vi "Update Properties in SysDef.vi"(8 "error in (no error)":errorcluster, 10 "Changed Properties":T1[](array[typedef]), 11 "Node Ptr":T2 format="%.0x") -> (0 "error out":errorcluster, 3 "Item Ref out":T2 format="%.0x")   [LabVIEW 2017]
doc: "Check which property value was changed and update that."
uses:
  SLSC EDS API/JSON parsing/property.ctl
  <vilib>/NI Veristand/Custom Device API/Custom Device API.lvlib
  Shared/Constants.vi
  Shared/SLSC EDS Shared.lvlib
  <vilib>/NI Veristand/Custom Device API/Set Item Property (Variant).vi
  <vilib>/NI Veristand/Custom Device API/Get Item Property (Variant).vi
  SLSC EDS API/JSON parsing/propertySysDefPage.ctl
  <vilib>/NI Veristand/Custom Device API/Custom Device Item Ref.ctl
panel:
  out "Properties":T1[](array[typedef])
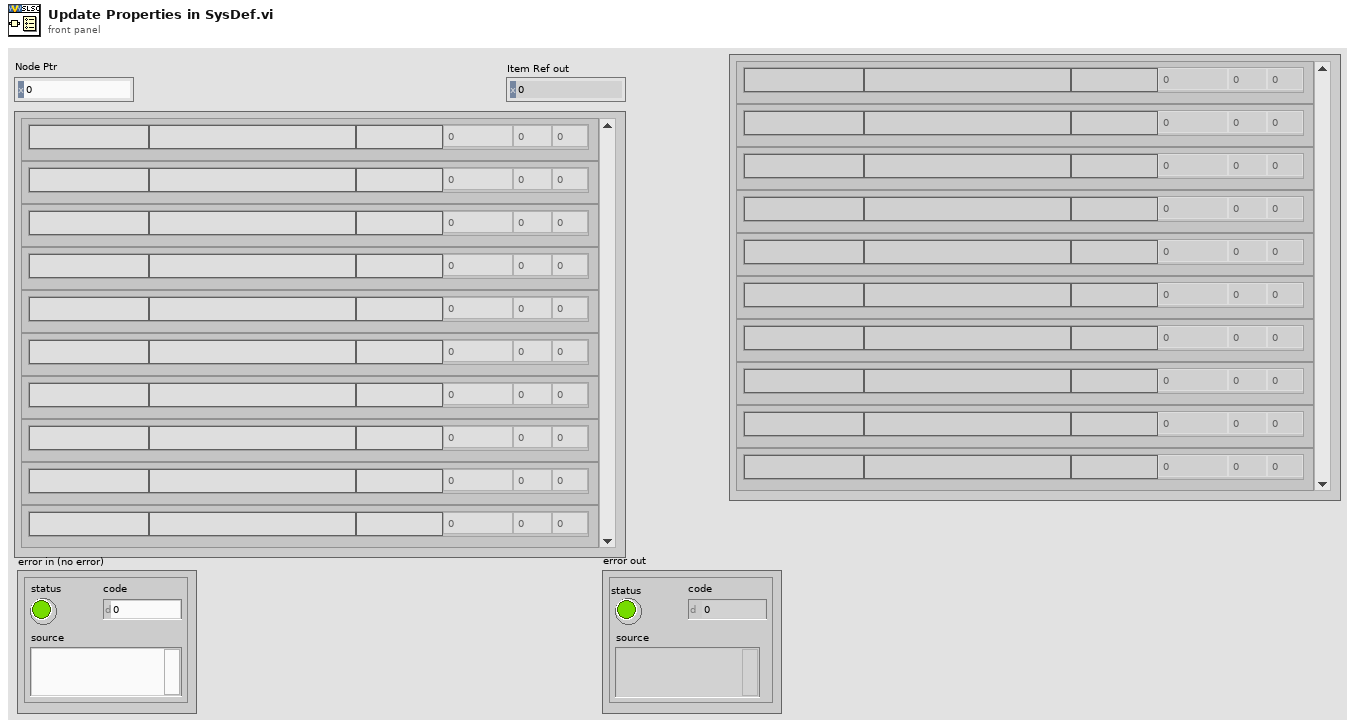
[diagram p1: front panel]
types:
  T1 = typedef "propertySysDefPage.ctl" = cluster{"name":string, "description-en":string, "dataType":string, "value":dbl, "min":dbl, "max":dbl}
  T2 = typedef "Custom Device API.lvlib/Custom Device Item Ref.ctl" = u64
  T3 = typedef "property.ctl" = cluster{"name":string, "description-en":string, "documentation-en":string, "dataType":string, "bitfield":string, "access":string, "scale":string, "value":variant, "min":variant, "max":variant, "default value":variant}
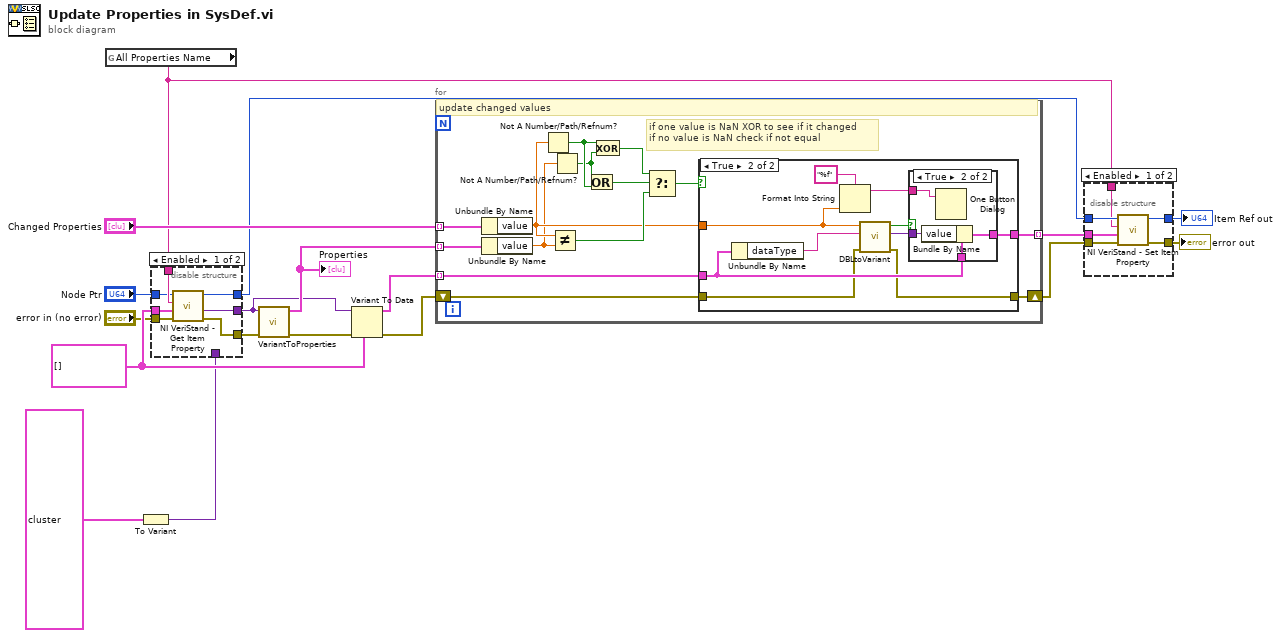
[diagram p0: block diagram]
diagram:
  w14 = T3[] [] ("properties")
  n1 = global read "Constants.vi" "All Properties Name"() -> (w10:string)
  n2 = To Variant(anything=T3[] [{"name"="NI.Debug.Alphabet", "description-en"="Constant string property", "documentation-en"="Constant string that returns the english alphabet", "dataType"="String", "bitfield"="", "access"="", "scale"="", "value"=variant(string "abcdefghijklmnopqrstuvwxyz"), "min"=variant, "max"=variant, "default value"=variant}, {"name"="NI.Debug.LED0Bool", "description-en"="one of 4 blue LEDs with Bool data type", "documentation-en"="towards back of module, under 2 caps, LED on far right", "dataType"="Bool", "bitfield"="DebugLeds/DebugLed0", "access"="WriteOnly", "scale"="", "value"=variant, "min"=variant, "max"=variant, "default value"=variant}, {"name"="NI.Debug.LED1Bool", "description-en"="one of 4 blue LEDs with Bool data type", "documentation-en"="towards back of module, under 2 caps, 2nd LED from the right", "dataType"="Bool", "bitfield"="DebugLeds/DebugLed1", "access"="ReadWrite", "scale"="", "value"=variant, "min"=variant, "max"=variant, "default value"=variant}, {"name"="NI.Debug.LED2Bool", "description-en"="one of 4 blue LEDs with Bool data type", "documentation-en"="towards back of module, under 2 caps, 2nd LED from the left", "dataType"="Bool", "bitfield"="DebugLeds/DebugLed2", "access"="ReadWrite", "scale"="", "value"=variant, "min"=variant, "max"=variant, "default value"=variant}, {"name"="NI.Debug.LED3Bool", "description-en"="one of 4 blue LEDs with Bool data type", "documentation-en"="towards back of module, under 2 caps, LED on far left", "dataType"="Bool", "bitfield"="DebugLeds/DebugLed3", "access"="ReadWrite", "scale"="", "value"=variant, "min"=variant, "max"=variant, "default value"=variant}, {"name"="NI.Debug.LED0Enum", "description-en"="one of 4 blue LEDs with Enum data type", "documentation-en"="towards back of module, under 2 caps, LED on far right", "dataType"="NI.LEDState", "bitfield"="DebugLeds/DebugLed0", "access"="WriteOnly", "scale"="", "value"=variant, "min"=variant, "max"=variant, "default value"=variant}, {"name"="NI.Debug.LED1Enum", "description-en"="one of 4 blue LEDs with Enum data type", "documentation-en"="towards back of module, under 2 caps, 2nd LED from the right", "dataType"="NI.LEDState", "bitfield"="DebugLeds/DebugLed1", "access"="ReadWrite", "scale"="", "value"=variant, "min"=variant, "max"=variant, "default value"=variant}, {"name"="NI.Debug.LED2Enum", "description-en"="one of 4 blue LEDs with Enum data type", "documentation-en"="towards back of module, under 2 caps, 2nd LED from the left", "dataType"="NI.LEDState", "bitfield"="DebugLeds/DebugLed2", "access"="ReadWrite", "scale"="", "value"=variant, "min"=variant, "max"=variant, "default value"=variant}, {"name"="NI.Debug.LED3Enum", "description-en"="one of 4 blue LEDs with Enum data type", "documentation-en"="towards back of module, under 2 caps, LED on far left", "dataType"="NI.LEDState", "bitfield"="DebugLeds/DebugLed3", "access"="ReadWrite", "scale"="", "value"=variant, "min"=variant, "max"=variant, "default value"=variant}, {"name"="NI.Scratchpad64.U64", "description-en"="use 64-bit Scratchpad as U64", "documentation-en"="Read write 64-bit scratchpad with U64 value", "dataType"="UInt64", "bitfield"="DebugScratch64/Scratch64", "access"="ReadWrite", "scale"="", "value"=variant, "min"=variant, "max"=variant, "default value"=variant}, {"name"="NI.Scratchpad64.I64", "description-en"="use 64-bit Scratchpad as I64", "documentation-en"="Read write 64-bit scratchpad with I64 value", "dataType"="Int64", "bitfield"="DebugScratch64/ScratchI64", "access"="ReadWrite", "scale"="", "value"=variant, "min"=variant, "max"=variant, "default value"=variant}, {"name"="NI.Scratchpad64.U32", "description-en"="use 64-bit Scratchpad as U32", "documentation-en"="Read write 64-bit scratchpad with U32 value", "dataType"="UInt32", "bitfield"="DebugScratch64/Scratch32", "access"="ReadWrite", "scale"="", "value"=variant, "min"=variant, "max"=variant, "default value"=variant}, {"name"="NI.Scratchpad64.I32", "description-en"="use 64-bit Scratchpad as I32", "documentation-en"="Read write 64-bit scratchpad with I32 value", "dataType"="Int32", "bitfield"="DebugScratch64/ScratchI32", "access"="ReadWrite", "scale"="", "value"=variant, "min"=variant, "max"=variant, "default value"=variant}, {"name"="NI.Scratchpad64.U16", "description-en"="use 64-bit Scratchpad as U16", "documentation-en"="Read write 64-bit scratchpad with U16 value", "dataType"="UInt32", "bitfield"="DebugScratch64/Scratch16", "access"="ReadWrite", "scale"="", "value"=variant, "min"=variant, "max"=variant, "default value"=variant}, {"name"="NI.Scratchpad64.I16", "description-en"="use 64-bit Scratchpad as I16", "documentation-en"="Read write 64-bit scratchpad with I16 value", "dataType"="Int32", "bitfield"="DebugScratch64/ScratchI16", "access"="ReadWrite", "scale"="", "value"=variant, "min"=variant, "max"=variant, "default value"=variant}, {"name"="NI.Scratchpad64.U8", "description-en"="use 64-bit Scratchpad as U8", "documentation-en"="Read write 64-bit scratchpad with U8 value", "dataType"="UInt32", "bitfield"="DebugScratch64/Scratch8", "access"="ReadWrite", "scale"="", "value"=variant, "min"=variant, "max"=variant, "default value"=variant}, {"name"="NI.Scratchpad64.I8", "description-en"="use 64-bit Scratchpad as I8", "documentation-en"="Read write 64-bit scratchpad with I8 value", "dataType"="Int32", "bitfield"="DebugScratch64/ScratchI8", "access"="ReadWrite", "scale"="", "value"=variant, "min"=variant, "max"=variant, "default value"=variant}, {"name"="NI.Scratchpad64.Bool", "description-en"="use 64-bit Scratchpad as Bool", "documentation-en"="Read write 64-bit scratchpad with Bool value", "dataType"="Bool", "bitfield"="DebugScratch64/ScratchBool", "access"="ReadWrite", "scale"="", "value"=variant, "min"=variant, "max"=variant, "default value"=variant}, {"name"="NI.Scratchpad32.U32", "description-en"="use 32-bit Scratchpad as U32", "documentation-en"="Read write 32-bit scratchpad with U32 value", "dataType"="UInt32", "bitfield"="DebugScratch32/Scratch32", "access"="ReadWrite", "scale"="", "value"=variant, "min"=variant, "max"=variant, "default value"=variant}, {"name"="NI.Scratchpad32.I32", "description-en"="use 32-bit Scratchpad as I32", "documentation-en"="Read write 32-bit scratchpad with I32 value", "dataType"="Int32", "bitfield"="DebugScratch32/ScratchI32", "access"="ReadWrite", "scale"="", "value"=variant, "min"=variant, "max"=variant, "default value"=variant}, {"name"="NI.Scratchpad32.U16", "description-en"="use 32-bit Scratchpad as U16", "documentation-en"="Read write 32-bit scratchpad with U16 value", "dataType"="UInt32", "bitfield"="DebugScratch32/Scratch16", "access"="ReadWrite", "scale"="", "value"=variant, "min"=variant, "max"=variant, "default value"=variant}, {"name"="NI.Scratchpad32.I16", "description-en"="use 32-bit Scratchpad as I16", "documentation-en"="Read write 32-bit scratchpad with I16 value", "dataType"="Int32", "bitfield"="DebugScratch32/ScratchI16", "access"="ReadWrite", "scale"="", "value"=variant, "min"=variant, "max"=variant, "default value"=variant}, {"name"="NI.Scratchpad32.U8", "description-en"="use 32-bit Scratchpad as U8", "documentation-en"="Read write 32-bit scratchpad with U8 value", "dataType"="UInt32", "bitfield"="DebugScratch32/Scratch8", "access"="ReadWrite", "scale"="", "value"=variant, "min"=variant, "max"=variant, "default value"=variant}, {"name"="NI.Scratchpad32.I8", "description-en"="use 32-bit Scratchpad as I8", "documentation-en"="Read write 32-bit scratchpad with I8 value", "dataType"="Int32", "bitfield"="DebugScratch32/ScratchI8", "access"="ReadWrite", "scale"="", "value"=variant, "min"=variant, "max"=variant, "default value"=variant}, {"name"="NI.Scratchpad32.Bool", "description-en"="use 32-bit Scratchpad as Bool", "documentation-en"="Read write 32-bit scratchpad with Bool value", "dataType"="Bool", "bitfield"="DebugScratch32/ScratchBool", "access"="ReadWrite", "scale"="", "value"=variant, "min"=variant, "max"=variant, "default value"=variant}, {"name"="NI.Scratchpad16.U16", "description-en"="use 16-bit Scratchpad as U16", "documentation-en"="Read write 16-bit scratchpad with U16 value", "dataType"="UInt32", "bitfield"="DebugScratch16/Scratch16", "access"="ReadWrite", "scale"="", "value"=variant, "min"=variant, "max"=variant, "default value"=variant}, {"name"="NI.Scratchpad16.I16", "description-en"="use 16-bit Scratchpad as I16", "documentation-en"="Read write 16-bit scratchpad with I16 value", "dataType"="Int32", "bitfield"="DebugScratch16/ScratchI16", "access"="ReadWrite", "scale"="", "value"=variant, "min"=variant, "max"=variant, "default value"=variant}, {"name"="NI.Scratchpad16.U8", "description-en"="use 16-bit Scratchpad as U8", "documentation-en"="Read write 16-bit scratchpad with U8 value", "dataType"="UInt32", "bitfield"="DebugScratch16/Scratch8", "access"="ReadWrite", "scale"="", "value"=variant, "min"=variant, "max"=variant, "default value"=variant}, {"name"="NI.Scratchpad16.I8", "description-en"="use 16-bit Scratchpad as I8", "documentation-en"="Read write 16-bit scratchpad with I8 value", "dataType"="Int32", "bitfield"="DebugScratch16/ScratchI8", "access"="ReadWrite", "scale"="", "value"=variant, "min"=variant, "max"=variant, "default value"=variant}, {"name"="NI.Scratchpad16.Bool", "description-en"="use 16-bit Scratchpad as Bool", "documentation-en"="Read write 16-bit scratchpad with Bool value", "dataType"="Bool", "bitfield"="DebugScratch16/ScratchBool", "access"="ReadWrite", "scale"="", "value"=variant, "min"=variant, "max"=variant, "default value"=variant}, {"name"="NI.Scratchpad8.U8", "description-en"="use 8-bit Scratchpad as U8", "documentation-en"="Read write 8-bit scratchpad with U8 value", "dataType"="UInt32", "bitfield"="DebugScratch8/Scratch8", "access"="ReadWrite", "scale"="", "value"=variant, "min"=variant, "max"=variant, "default value"=variant}, {"name"="NI.Scratchpad8.I8", "description-en"="use 8-bit Scratchpad as I8", "documentation-en"="Read write 8-bit scratchpad with I8 value", "dataType"="Int32", "bitfield"="DebugScratch8/ScratchI8", "access"="ReadWrite", "scale"="", "value"=variant, "min"=variant, "max"=variant, "default value"=variant}, {"name"="NI.Scratchpad8.Bool", "description-en"="use 8-bit Scratchpad as Bool", "documentation-en"="Read write 8-bit scratchpad with Bool value", "dataType"="Bool", "bitfield"="DebugScratch8/ScratchBool", "access"="ReadWrite", "scale"="", "value"=variant, "min"=variant, "max"=variant, "default value"=variant}, {"name"="NI.Debug.ScratchU32.Min10", "description-en"="", "documentation-en"="", "dataType"="UInt32", "bitfield"="DebugScratch32/Scratch32", "access"="ReadWrite", "scale"="", "value"=variant, "min"=variant(u64 10), "max"=variant, "default value"=variant}, {"name"="NI.Debug.ScratchU32.Max10", "description-en"="", "documentation-en"="", "dataType"="UInt32", "bitfield"="DebugScratch32/Scratch32", "access"="ReadWrite", "scale"="", "value"=variant, "min"=variant, "max"=variant(u64 10), "default value"=variant}, {"name"="NI.Debug.ScratchU32.Min10Max20", "description-en"="", "documentation-en"="", "dataType"="UInt32", "bitfield"="DebugScratch32/Scratch32", "access"="ReadWrite", "scale"="", "value"=variant, "min"=variant(u64 10), "max"=variant(u64 20), "default value"=variant}, {"name"="NI.Debug.ScratchI32.Strict4", "description-en"="", "documentation-en"="", "dataType"="Int32", "bitfield"="DebugScratch32/ScratchI32", "access"="ReadWrite", "scale"="TableStrict4Elements", "value"=variant, "min"=variant, "max"=variant, "default value"=variant}, {"name"="NI.Debug.ScratchI32.Strict12", "description-en"="", "documentation-en"="", "dataType"="Int32", "bitfield"="DebugScratch32/ScratchI32", "access"="ReadWrite", "scale"="TableStrict12Elements", "value"=variant, "min"=variant(i64 -2), "max"=variant(i64 -1), "default value"=variant}, {"name"="NI.Debug.ScratchU32.UInt32.Times2Plus2", "description-en"="", "documentation-en"="", "dataType"="UInt32", "bitfield"="DebugScratch32/Scratch32", "access"="ReadWrite", "scale"="Times2Plus2", "value"=variant, "min"=variant, "max"=variant, "default value"=variant}, {"name"="NI.Debug.ScratchU32.Double", "description-en"="", "documentation-en"="", "dataType"="Double", "bitfield"="DebugScratch32/Scratch32", "access"="ReadWrite", "scale"="", "value"=variant, "min"=variant, "max"=variant, "default value"=variant}, {"name"="NI.Debug.ScratchU32.Double.LinearDivideBy8.Min7Max10", "description-en"="", "documentation-en"="", "dataType"="Double", "bitfield"="DebugScratch32/Scratch32", "access"="ReadWrite", "scale"="LinearDivideBy8", "value"=variant, "min"=variant(ext 7.0), "max"=variant(ext 10.0), "default value"=variant}, {"name"="NI.Debug.ScratchU32.Double.PolynomialThermocouple", "description-en"="", "documentation-en"="", "dataType"="Double", "bitfield"="DebugScratch32/Scratch32", "access"="ReadWrite", "scale"="PolynomialThermocouple", "value"=variant, "min"=variant(ext 0.0), "max"=variant(ext 760.0), "default value"=variant}, {"name"="NI.Debug.ScratchU32.Double.TableStrict", "description-en"="", "documentation-en"="", "dataType"="Double", "bitfield"="DebugScratch32/Scratch32", "access"="ReadWrite", "scale"="TableStrict", "value"=variant, "min"=variant, "max"=variant, "default value"=variant}, {"name"="NI.Debug.ScratchU32.Int32.TableStrict", "description-en"="", "documentation-en"="", "dataType"="Int32", "bitfield"="DebugScratch32/Scratch32", "access"="ReadWrite", "scale"="TableStrict", "value"=variant, "min"=variant(i64 -2), "max"=variant(u64 8), "default value"=variant}, {"name"="NI.Debug.ScratchU32.Double.TableInterpolate", "description-en"="", "documentation-en"="", "dataType"="Double", "bitfield"="DebugScratch32/Scratch32", "access"="ReadWrite", "scale"="TableInterpolate", "value"=variant, "min"=variant, "max"=variant, "default value"=variant}, {"name"="NI.Debug.ScratchU32.Double.TableRound", "description-en"="", "documentation-en"="", "dataType"="Double", "bitfield"="DebugScratch32/Scratch32", "access"="ReadWrite", "scale"="TableRound", "value"=variant, "min"=variant, "max"=variant, "default value"=variant}, {"name"="NI.Debug.ScratchBool.InvertBoolean", "description-en"="", "documentation-en"="", "dataType"="Bool", "bitfield"="DebugScratch64/ScratchBool", "access"="ReadWrite", "scale"="InvertBoolean", "value"=variant, "min"=variant, "max"=variant, "default value"=variant}, {"name"="NI.Debug.ScratchBool.TableStrictTrueFalse", "description-en"="", "documentation-en"="", "dataType"="Bool", "bitfield"="DebugScratch64/Scratch64", "access"="ReadWrite", "scale"="TableStrictTrueFalse", "value"=variant, "min"=variant, "max"=variant, "default value"=variant}, {"name"="NI.Debug.ScratchBool.TableStrictFalse", "description-en"="", "documentation-en"="", "dataType"="Bool", "bitfield"="DebugScratch64/Scratch64", "access"="ReadWrite", "scale"="TableStrictFalse", "value"=variant, "min"=variant, "max"=variant, "default value"=variant}, {"name"="NI.Debug.ScratchBool.TableStrictTrue", "description-en"="", "documentation-en"="", "dataType"="Bool", "bitfield"="DebugScratch64/Scratch64", "access"="ReadWrite", "scale"="TableStrictTrue", "value"=variant, "min"=variant, "max"=variant, "default value"=variant}, {"name"="NI.GreenLED0", "description-en"="one of 3 tri-colored LEDs (red/green/amber), controls green", "documentation-en"="towards front of module, at the top, left LED", "dataType"="Bool", "bitfield"="FrontPanelLeds/LedGreen0Enable", "access"="WriteOnly", "scale"="", "value"=variant, "min"=variant, "max"=variant, "default value"=variant}, {"name"="NI.GreenLED1", "description-en"="one of 3 tri-colored LEDs (red/green/amber), controls green", "documentation-en"="towards front of module, at the top, center LED", "dataType"="Bool", "bitfield"="FrontPanelLeds/LedGreen1Enable", "access"="WriteOnly", "scale"="", "value"=variant, "min"=variant, "max"=variant, "default value"=variant}, {"name"="NI.GreenLED2", "description-en"="one of 3 tri-colored LEDs (red/green/amber), controls green", "documentation-en"="towards front of module, at the top, right LED", "dataType"="Bool", "bitfield"="FrontPanelLeds/LedGreen2Enable", "access"="WriteOnly", "scale"="", "value"=variant, "min"=variant, "max"=variant, "default value"=variant}, {"name"="NI.RedLED0", "description-en"="one of 3 tri-colored LEDs (red/green/amber), controls red", "documentation-en"="towards front of module, at the top, left LED", "dataType"="Bool", "bitfield"="FrontPanelLeds/LedRed0Enable", "access"="WriteOnly", "scale"="", "value"=variant, "min"=variant, "max"=variant, "default value"=variant}, {"name"="NI.RedLED1", "description-en"="one of 3 tri-colored LEDs (red/green/amber), controls red", "documentation-en"="towards front of module, at the top, center LED", "dataType"="Bool", "bitfield"="FrontPanelLeds/LedRed1Enable", "access"="WriteOnly", "scale"="", "value"=variant, "min"=variant, "max"=variant, "default value"=variant}, {"name"="NI.RedLED2", "description-en"="one of 3 tri-colored LEDs (red/green/amber), controls red", "documentation-en"="towards front of module, at the top, right LED", "dataType"="Bool", "bitfield"="FrontPanelLeds/LedRed2Enable", "access"="WriteOnly", "scale"="", "value"=variant, "min"=variant, "max"=variant, "default value"=variant}, {"name"="NI.EventCounter0", "description-en"="", "documentation-en"="", "dataType"="UInt32", "bitfield"="EventCounter0/DelayInMilliseconds", "access"="ReadWrite", "scale"="", "value"=variant, "min"=variant, "max"=variant(u64 255), "default value"=variant}, {"name"="NI.EventCounter1", "description-en"="", "documentation-en"="", "dataType"="UInt32", "bitfield"="EventCounter1/DelayInMilliseconds", "access"="ReadWrite", "scale"="", "value"=variant, "min"=variant, "max"=variant(u64 255), "default value"=variant}, {"name"="NI.EventCounter2", "description-en"="", "documentation-en"="", "dataType"="UInt32", "bitfield"="EventCounter2/DelayInMilliseconds", "access"="ReadWrite", "scale"="", "value"=variant, "min"=variant, "max"=variant(u64 255), "default value"=variant}, {"name"="NI.EventCounter3", "description-en"="", "documentation-en"="", "dataType"="UInt32", "bitfield"="EventCounter3/DelayInMilliseconds", "access"="ReadWrite", "scale"="", "value"=variant, "min"=variant, "max"=variant(u64 255), "default value"=variant}, {"name"="NI.EventCounter0.DelayInMs", "description-en"="", "documentation-en"="", "dataType"="UInt32", "bitfield"="EventCounter0/DelayInMilliseconds", "access"="ReadWrite", "scale"="", "value"=variant, "min"=variant, "max"=variant(u64 255), "default value"=variant}, {"name"="NI.EventCounter1.DelayInMs", "description-en"="", "documentation-en"="", "dataType"="UInt32", "bitfield"="EventCounter1/DelayInMilliseconds", "access"="ReadWrite", "scale"="", "value"=variant, "min"=variant, "max"=variant(u64 255), "default value"=variant}, {"name"="NI.EventCounter2.DelayInMs", "description-en"="", "documentation-en"="", "dataType"="UInt32", "bitfield"="EventCounter2/DelayInMilliseconds", "access"="ReadWrite", "scale"="", "value"=variant, "min"=variant, "max"=variant(u64 255), "default value"=variant}, {"name"="NI.EventCounter3.DelayInMs", "description-en"="", "documentation-en"="", "dataType"="UInt32", "bitfield"="EventCounter3/DelayInMilliseconds", "access"="ReadWrite", "scale"="", "value"=variant, "min"=variant, "max"=variant(u64 255), "default value"=variant}, {"name"="NI.EventCounter0.DelayInSec", "description-en"="", "documentation-en"="", "dataType"="Double", "bitfield"="EventCounter0/DelayInMilliseconds", "access"="ReadWrite", "scale"="LinearMillisecondToSecond", "value"=variant, "min"=variant(ext 0.0), "max"=variant(ext 0.255), "default value"=variant}, {"name"="NI.EventCounter1.DelayInSec", "description-en"="", "documentation-en"="", "dataType"="Double", "bitfield"="EventCounter1/DelayInMilliseconds", "access"="ReadWrite", "scale"="LinearMillisecondToSecond", "value"=variant, "min"=variant(ext 0.0), "max"=variant(ext 0.255), "default value"=variant}, {"name"="NI.EventCounter2.DelayInSec", "description-en"="", "documentation-en"="", "dataType"="Double", "bitfield"="EventCounter2/DelayInMilliseconds", "access"="ReadWrite", "scale"="LinearMillisecondToSecond", "value"=variant, "min"=variant(ext 0.0), "max"=variant(ext 0.255), "default value"=variant}, {"name"="NI.EventCounter3.DelayInSec", "description-en"="", "documentation-en"="", "dataType"="Double", "bitfield"="EventCounter3/DelayInMilliseconds", "access"="ReadWrite", "scale"="LinearMillisecondToSecond", "value"=variant, "min"=variant(ext 0.0), "max"=variant(ext 0.255), "default value"=variant}, {"name"="NI.EventCounter0.DelayEnum", "description-en"="", "documentation-en"="", "dataType"="NI.EventDelay", "bitfield"="EventCounter0/DelayInMilliseconds", "access"="ReadWrite", "scale"="", "value"=variant, "min"=variant, "max"=variant, "default value"=variant}, {"name"="NI.EventCounter1.DelayEnum", "description-en"="", "documentation-en"="", "dataType"="NI.EventDelay", "bitfield"="EventCounter1/DelayInMilliseconds", "access"="ReadWrite", "scale"="", "value"=variant, "min"=variant, "max"=variant, "default value"=variant}, {"name"="NI.EventCounter2.DelayEnum", "description-en"="", "documentation-en"="", "dataType"="NI.EventDelay", "bitfield"="EventCounter2/DelayInMilliseconds", "access"="ReadWrite", "scale"="", "value"=variant, "min"=variant, "max"=variant, "default value"=variant}, {"name"="NI.EventCounter3.DelayEnum", "description-en"="", "documentation-en"="", "dataType"="NI.EventDelay", "bitfield"="EventCounter3/DelayInMilliseconds", "access"="ReadWrite", "scale"="", "value"=variant, "min"=variant, "max"=variant, "default value"=variant}] ("properties")) -> (Variant=w1:variant)
  n3 = disable-structure shown="Enabled" {
    disable-tunnel: [w25 w27] -> w15
    disable-tunnel: w14 -> [w24 _]
    disable-tunnel: [w23 _] -> w11
    disable-tunnel: w10 -> [w22 _]
    disable-tunnel: "Node Ptr" -> [w21 _]
    disable-tunnel: "error in (no error)" -> [w20 w26]
    disable-tunnel: [w19 w26] -> w3
    disable-tunnel: w1 -> [_ w27]
    frame Enabled {
      n4 = call-poly <vilib>:"NI VeriStand - Get Item Property.vi"("error in (no error)"=w20, "Default Value"=w24, "Property Name"=w22, "Item Ref in"=w21) -> ("error out"=w19:errorcluster, "Value"=w25:variant, "Item Ref out"=w23:T2)  [unwired: 4 in, 1 out]
    }
    frame Disabled {
    }
  }
  n5 = call "VariantToProperties.vi"("error in (no error)"=w3, "Variant"=w15) -> ("error out"=w16:errorcluster, "Properties"=w17:T1[])  [unwired: 8 in]
  "Properties" <- w17
  n6 = Variant To Data(error in=w16, type=w14, Variant=w15) -> (data=w13:T3[], error out=w12:errorcluster)
  n7 = for {
    tunnel: "Changed Properties" -> [w41] mode=indexing
    tunnel: w17 -> [w40] mode=indexing
    tunnel: w13 -> [w39] mode=indexing
    shift-right: [w37] -> w8
    shift-left: w12 -> [w38]
    tunnel: [w36] -> w9 mode=indexing
    # "if one value is NaN XOR to see if it changed\nif no value is NaN check if not equal"
    # "update changed values"
    n8 = Unbundle By Name(w41) -> ("value"=w29:dbl)
    n9 = Unbundle By Name(w40) -> ("value"=w28:dbl)
    n10 = Not A Number/Path/Refnum?(number/path/refnum=w29) -> (NaN/Path/Refnum?=w33:bool)
    n11 = Not Equal?(x=w29, y=w28) -> (x != y?=w31:bool)
    n12 = Not A Number/Path/Refnum?(number/path/refnum=w28) -> (NaN/Path/Refnum?=w32:bool)
    n13 = Or(x=w32, y=w33) -> (x .or. y?=w34:bool)
    n14 = Exclusive Or(1:w32, 2:w33) -> (0:w35:bool)
    n15 = Select(t=w35, s=w34, f=w31) -> (s? t:f=w30:bool)
    n16 = case shown="True" w30 {
      tunnel: w29 -> [_ w46]
      tunnel: w39 -> [w42 w52]
      tunnel: w38 -> [w43 w51]
      tunnel: [w43 w50] -> w37
      tunnel: [w42 w48] -> w36
      frame False {
      }
      frame True {
        n17 = Unbundle By Name(w52) -> ("dataType"=w44:string)
        n18 = Format Into String(format string="%f", w46) -> (resulting string=w45:string)  [unwired: 2 in, 1 out]
        n19 = call "DBLtoVariant.vi"("error in"=w51, "dataType"=w44, "data"=w46) -> ("error out"=w50:errorcluster, "variant out"=w53:variant, "valid?"=w49:bool)  [unwired: 6 in]
        n20 = case shown="True" w49 {
          tunnel: w53 -> [_ w58]
          tunnel: w52 -> [w54 w57]
          tunnel: [w54 w56] -> w48
          tunnel: w45 -> [_ w55]
          frame False {
          }
          frame True {
            n21 = Bundle By Name(cluster=w57, "value"=w58) -> (w56:T3)
            n22 = One Button Dialog(message=w55) -> ()  [unwired: 1 in, 1 out]
          }
        }
      }
    }
  }
  n23 = disable-structure shown="Enabled" {
    disable-tunnel: w11 -> [w64 _]
    disable-tunnel: w10 -> [w63 _]
    disable-tunnel: w9 -> [w62 _]
    disable-tunnel: w8 -> [w61 w65]
    disable-tunnel: [w60 w65] -> w7
    disable-tunnel: [w59 _] -> w6
    frame Enabled {
      n24 = call-poly <vilib>:"NI VeriStand - Set Item Property.vi"("error in (no error)"=w61, "Value"=w62, "Property Name"=w63, "Item Ref in"=w64) -> ("error out"=w60:errorcluster, "Item Ref out"=w59:T2)  [unwired: 5 in, 1 out]
    }
    frame Disabled {
    }
  }
  "error out" <- w7
  "Item Ref out" <- w6
